vi "Create Parameter For Each Word.vi"(8 "error in":errorcluster, 11 "number of words":u16) -> (0 "error out":errorcluster, 3 "parameters":T2(array[cluster]))   [LabVIEW 2020]
uses:
  Parameter Definition.ctl
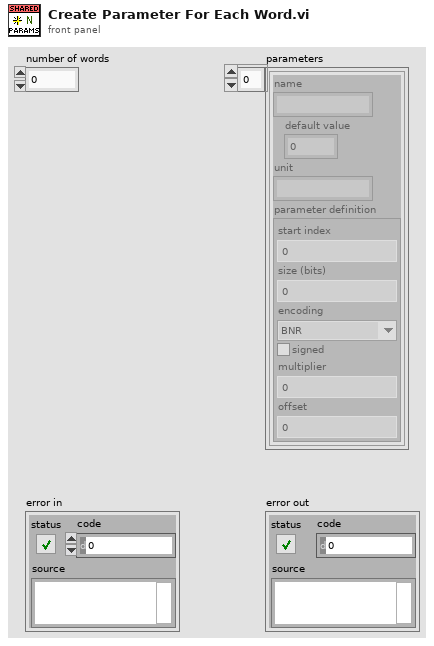
[diagram p1: front panel]
types:
  T1 = typedef "Parameter Definition.ctl" = cluster{"start index":i32, "size (bits)":i32, "encoding":enum16{"BNR", "BCD", "Discrete"}, "signed":bool, "multiplier":dbl, "offset":dbl}
  T2 = cluster{"name":string, "default value":dbl, "unit":string, "parameter definition":T1}[]
  T3 = cluster{"name":string, "default value":dbl, "unit":string, "parameter definition":T1}
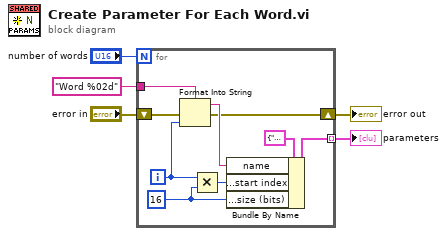
[diagram p0: block diagram]
diagram:
  n1 = for {
    N: "number of words" -> [_]
    tunnel: [w7] -> w3 mode=indexing
    shift-right: [w8] -> w5
    shift-left: "error in" -> [w9]
    tunnel: "Word %02d" ("format string") -> [w6]
    i -> [w12]
    w11 = 16 ("y")
    n2 = Format Into String(format string=w6, error in=w9, w12) -> (resulting string=w14:string, error out=w8:errorcluster)  [unwired: 1 in]
    n3 = Multiply(x=w12, y=w11) -> (x*y=w13:i32)
    n4 = Bundle By Name(cluster=T3 {"name"="", "default value"=1.0, "unit"="", "parameter definition"={"start index"=0, "size (bits)"=16, "encoding"=enum."BNR", "signed"=FALSE, "multiplier"=1.0, "offset"=0.0}} ("definition with default value"), "name"=w14, "parameter definition.start index"=w13, "parameter definition.size (bits)"=w11) -> (w7:T3)
  }
  "error out" <- w5
  "parameters" <- w3
